vi "Unique Path Name.vi"(3 "error in":errorcluster, 5 "Base Path":path) -> (0 "error out":errorcluster, 1 "Run Number":i32, 2 "Unique Path":path)   [LabVIEW 2014]
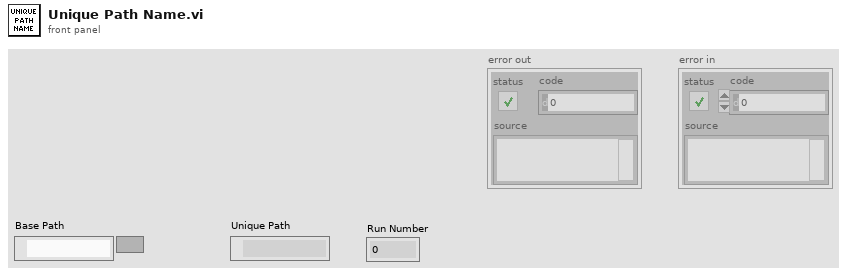
[diagram p1: front panel]
types:
  T1 = enum16{"open", "replace", "create", "open or create", "replace or create", "replace or create with confirmation"}
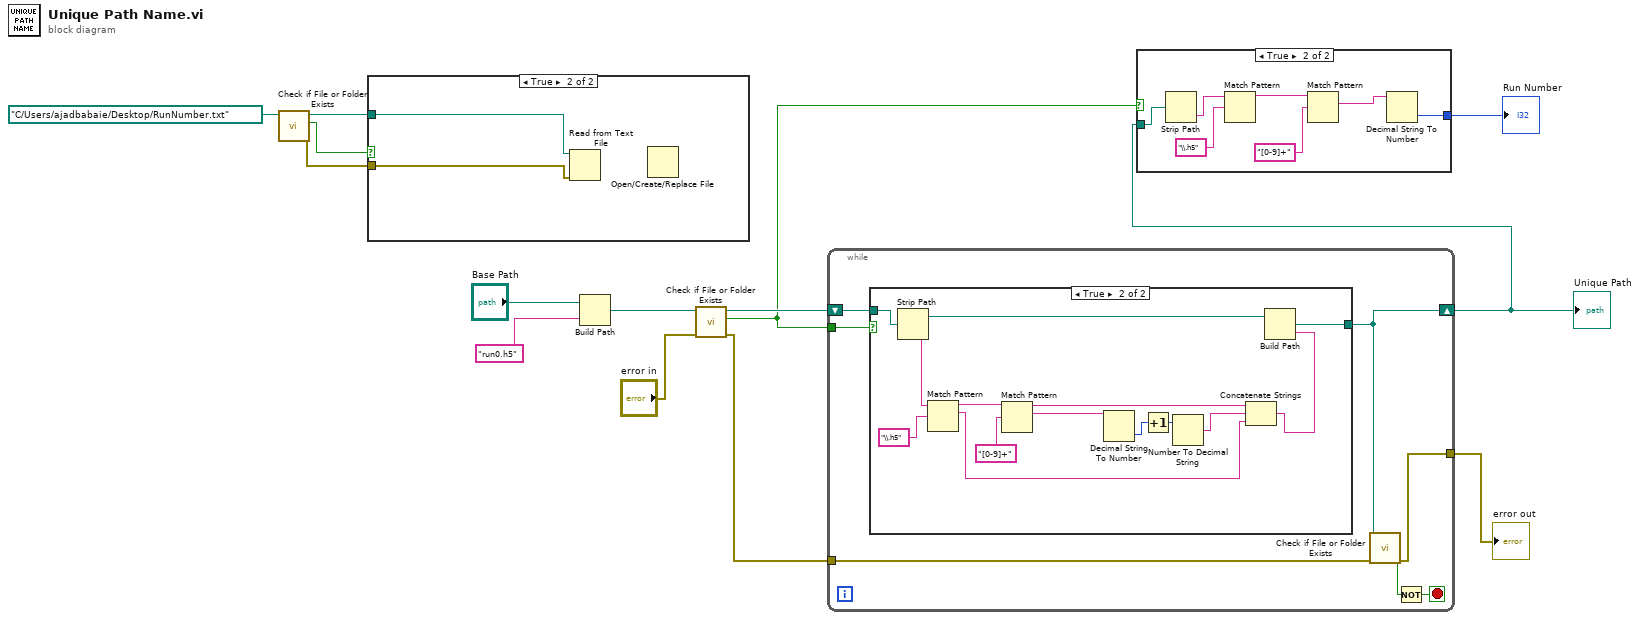
[diagram p0: block diagram]
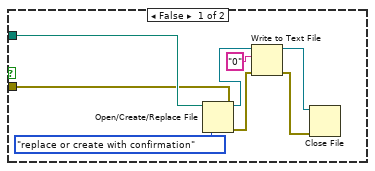
[diagram p2: hidden frame]
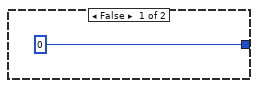
[diagram p3: hidden frame]
diagram:
  n1 = call <vilib>:"Check if File or Folder Exists.vi"("path"=path "C:/Users/ajadbabaie/Desktop/RunNumber.txt") -> ("error out"=w2:errorcluster, "file or folder exists?"=w1:bool, "dup path"=w3:path)  [unwired: 8 in]
  n2 = case shown="True" w1 {
    tunnel: w3 -> [w22 w23]
    tunnel: w2 -> [w20 w24]
    frame False {
      n3 = Open/Create/Replace File(file path (use dialog)=w22, error in=w20, operation (0:open)=T1."replace or create with confirmation") -> (refnum out=w18:refnum<file>, error out=w17:errorcluster)  [unwired: 3 in, 1 out]
      n4 = Write to Text File(file (use dialog)=w18, text="0", error in=w17) -> (refnum out=w15:refnum<file>, error out=w16:errorcluster)  [unwired: 1 in, 1 out]
      n5 = Close File(refnum=w15, error in=w16) -> ()  [unwired: 2 out]
    }
    frame True {
      n6 = Read from Text File(file (use dialog)=w23, error in=w24) -> ()  [unwired: 2 in, 4 out]
      n7 = Open/Create/Replace File() -> ()  [unwired: 6 in, 3 out]
    }
  }
  n8 = Build Path(base path="Base Path", name or relative path="run0.h5") -> (appended path=w6:path)
  n9 = call <vilib>:"Check if File or Folder Exists.vi"("error in (no error)"="error in", "path"=w6) -> ("error out"=w13:errorcluster, "file or folder exists?"=w5:bool, "dup path"=w14:path)  [unwired: 7 in]
  n10 = while {
    shift-right: [w30] -> w9
    shift-left: w14 -> [w31]
    tunnel: w5 -> [w25]
    tunnel: w13 -> [w27]
    tunnel: [w26] -> w12
    stop <- w28 stop-if-true
    n11 = case shown="True" w25 {
      tunnel: [w32 w44] -> w30
      tunnel: w31 -> [w32 w46]
      frame False {
      }
      frame True {
        n12 = Strip Path(path=w46) -> (stripped path=w45:path, name=w38:string)
        n13 = Match Pattern(string=w38, regular expression="\\.h5") -> (before substring=w34:string, match substring=w33:string)  [unwired: 1 in, 2 out]
        n14 = Match Pattern(string=w34, regular expression="[0-9]+") -> (before substring=w42:string, match substring=w40:string)  [unwired: 1 in, 2 out]
        n15 = Decimal String To Number(string=w40) -> (number=w37:i32)  [unwired: 2 in, 1 out]
        n16 = Increment(x=w37) -> (x+1=w36:i32)
        n17 = Number To Decimal String(number=w36) -> (decimal integer string=w35:string)  [unwired: 1 in]
        n18 = Concatenate Strings(w42, w35, w33) -> (w41:string)
        n19 = Build Path(base path=w45, name or relative path=w41) -> (appended path=w44:path)
      }
    }
    n20 = call <vilib>:"Check if File or Folder Exists.vi"("error in (no error)"=w27, "path"=w30) -> ("error out"=w26:errorcluster, "file or folder exists?"=w29:bool)  [unwired: 7 in, 1 out]
    n21 = Not(x=w29) -> (.not. x?=w28:bool)
  }
  "Unique Path" <- w9
  "error out" <- w12
  n22 = case shown="True" w5 {
    tunnel: [0 w51] -> w10
    tunnel: w9 -> [_ w54]
    frame False {
    }
    frame True {
      n23 = Strip Path(path=w54) -> (name=w49:string)  [unwired: 1 out]
      n24 = Match Pattern(string=w49, regular expression="\\.h5") -> (before substring=w48:string)  [unwired: 1 in, 3 out]
      n25 = Match Pattern(string=w48, regular expression="[0-9]+") -> (match substring=w52:string)  [unwired: 1 in, 3 out]
      n26 = Decimal String To Number(string=w52) -> (number=w51:i32)  [unwired: 2 in, 1 out]
    }
  }
  "Run Number" <- w10
